vi "DAC Configure FP View.vi"(8 "error in":errorcluster, 11 "DAC Inverter in":refnum<class "DAC Inverter.lvclass">) -> (0 "error out":errorcluster, 3 "DAC Inverter out":refnum<class "DAC Inverter.lvclass">)   [LabVIEW 2019, in "DAC.lvlib" / "DAC Inverter.lvclass"]
uses:
  DAC Inverter.lvclass
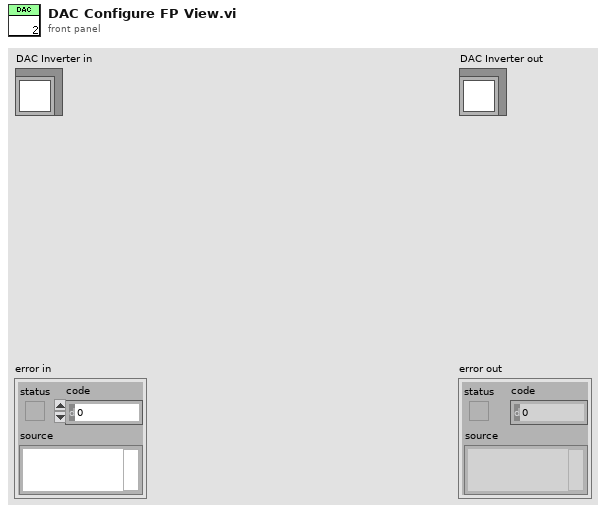
[diagram p1: front panel]
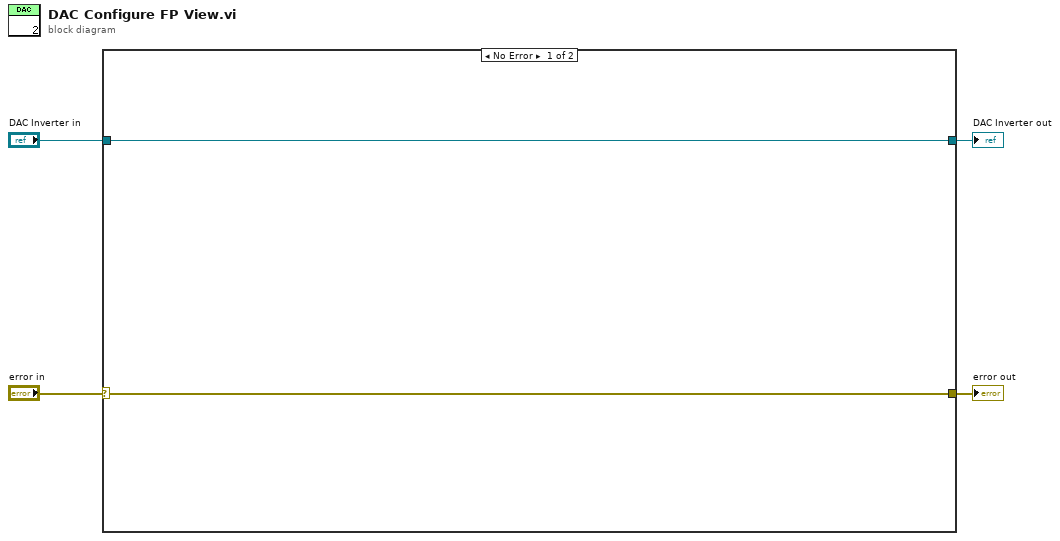
[diagram p0: block diagram]
diagram:
  n1 = case shown="No Error" "error in" {
    selector: "error in" -> [w5 w8]
    tunnel: [w5 w8] -> w1
    tunnel: [w6 w7] -> w2
    tunnel: "DAC Inverter in" -> [w6 w7]
    frame No Error {
    }
    frame Error {
    }
  }
  "error out" <- w1
  "DAC Inverter out" <- w2
